vi "PID.vi"(8 "error in (no error)":errorcluster, 11 "PID Loop in":refnum<class "PID Loop.lvclass">) -> (0 "error out":errorcluster, 3 "PID Loop out":refnum<class "PID Loop.lvclass">)   [LabVIEW 2024, in "PID Loop.lvlib" / "PID Loop.lvclass"]
uses:
  PID Loop.lvclass
  PID Loop.lvclass/PID Loop.ctl
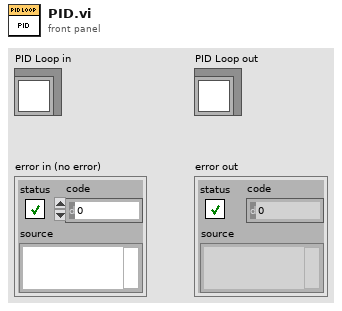
[diagram p1: front panel]
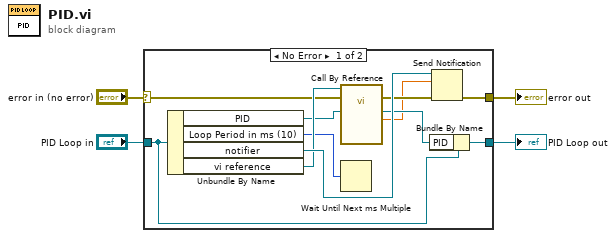
[diagram p0: block diagram]
diagram:
  n1 = case shown="No Error" "error in (no error)" {
    selector: "error in (no error)" -> [w6 w17]
    tunnel: [w14 w17] -> w3
    tunnel: [w10 w16] -> w1
    tunnel: "PID Loop in" -> [w11 w16]
    frame No Error {
      n2 = Unbundle By Name(w11) -> ("PID"=w9:refnum<class "PID.lvclass">, "Loop Period in ms (10)"=w5:u32, "notifier"=w15:refnum<notifier>, "vi reference"=w13:refnum<vi>)
      n3 = call-by-ref "?"(reference=w13, error in=w6, "PID in"=w9) -> (error out=w12:errorcluster, "output"=w7:dbl, "PID out"=w8:refnum<class "PID.lvclass">)  [unwired: 8 in, 2 out]
      n4 = Wait Until Next ms Multiple(millisecond multiple=w5) -> ()  [unwired: 1 out]
      n5 = Bundle By Name(cluster=w11, "PID"=w8) -> (w10:refnum<class "PID Loop.lvclass">)
      n6 = Send Notification(notification=w7, notifier=w15, error in (no error)=w12) -> (error out=w14:errorcluster)  [unwired: 1 out]
    }
    frame Error {
    }
  }
  "error out" <- w3
  "PID Loop out" <- w1
